vi "Close API Reference.vi"(8 "error in (no error)":errorcluster, 11 "Execution API in":refnum<class "Execution API.lvclass">) -> (0 "error out":errorcluster)   [LabVIEW 2020, in "Execution API.lvclass"]
doc: "Closes the API reference. Please note that any Event Registrations obtained from the Register for Events.vi will need to be unregistered for."
uses:
  Execution API.lvclass
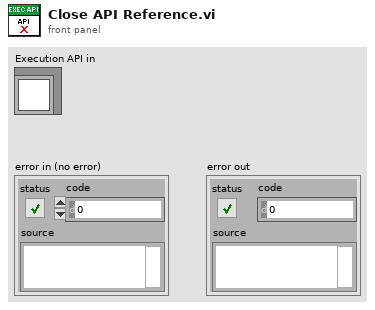
[diagram p1: front panel]
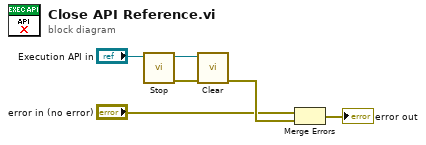
[diagram p0: block diagram]
diagram:
  n1 = call-dynamic "Stop.vi"("Process In"="Execution API in") -> ("error out"=w4:errorcluster, "Process Out"=w5:refnum<class "Execution API.lvclass">)  [unwired: 8 in, 1 out]
  n2 = call-dynamic "Clear.vi"("error in (no error)"=w4, "Execution API In"=w5) -> ("error out"=w6:errorcluster)  [unwired: 8 in, 1 out]
  n3 = Merge Errors("error in (no error)", w6) -> (→"error out":errorcluster)
